vi "ROS_Master_Main.vi"(11 "ROS_Master in":refnum<class "ROS_Master.lvclass">) -> ()   [LabVIEW 2012, in "ROS_Master.lvclass"]
uses:
  <userlib>/ROSforLV/ROS/Code/ROS_Master/ROS_Master.lvclass
  <userlib>/ROSforLV/ROS/Code/ROS_Master/ROS_Master.lvclass/ROS_Master.ctl
  <userlib>/ROSforLV/ROS/Code/_ROSDefinition.vi
panel:
  in  "Port":u32=11311
  in  "stop":bool
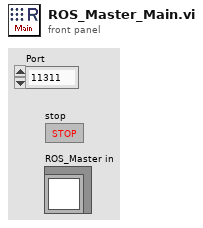
[diagram p1: front panel]
types:
  T1 = cluster{"Caller ID":string, "IP":string, "Msg Type":string, "Direction":enum16{"Publisher", "Subscriber"}, "Topic":string}
  T2 = cluster{"value":string, "value":string, "value":string}
  T3 = cluster{"Service":string, "Service IP":string, "Caller IP":string, "Caller ID":string}[]
  T4 = cluster{"Service":string, "Service IP":string, "Caller IP":string, "Caller ID":string}
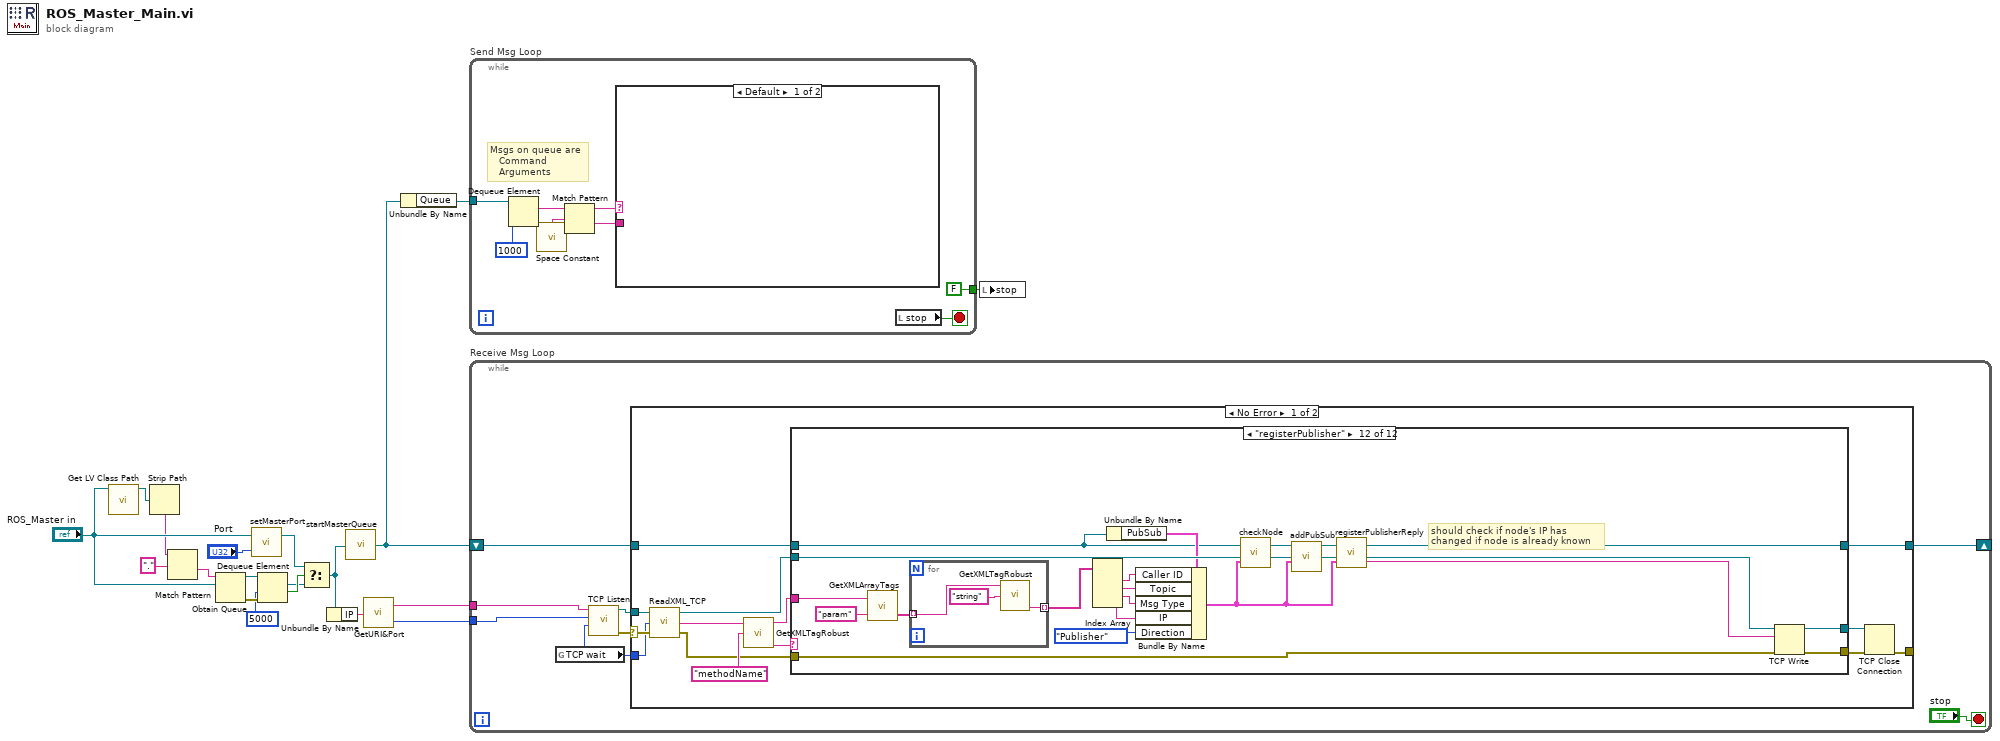
[diagram p0: block diagram]
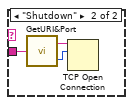
[diagram p2: hidden frame]
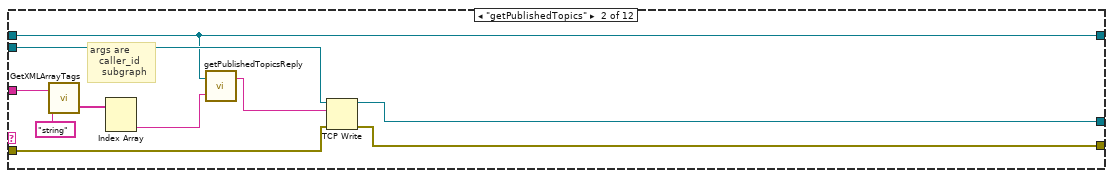
[diagram p4: hidden frame]
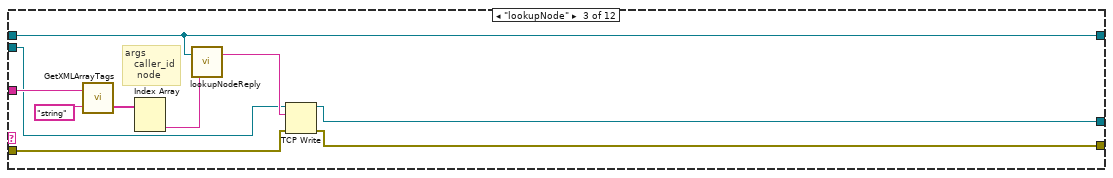
[diagram p5: hidden frame]
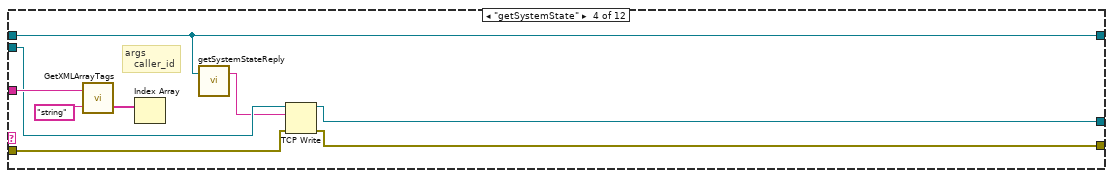
[diagram p6: hidden frame]
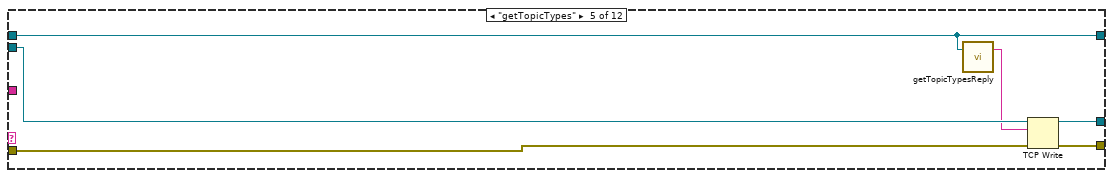
[diagram p7: hidden frame]
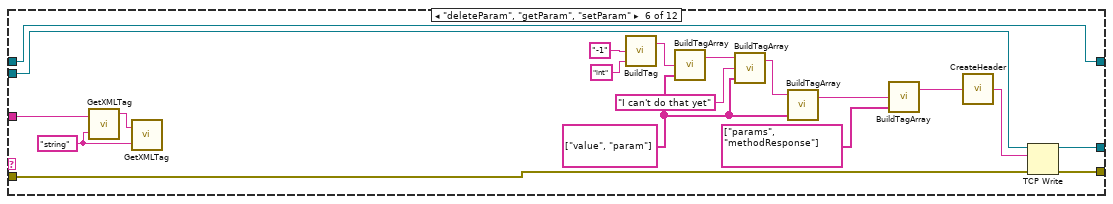
[diagram p8: hidden frame]
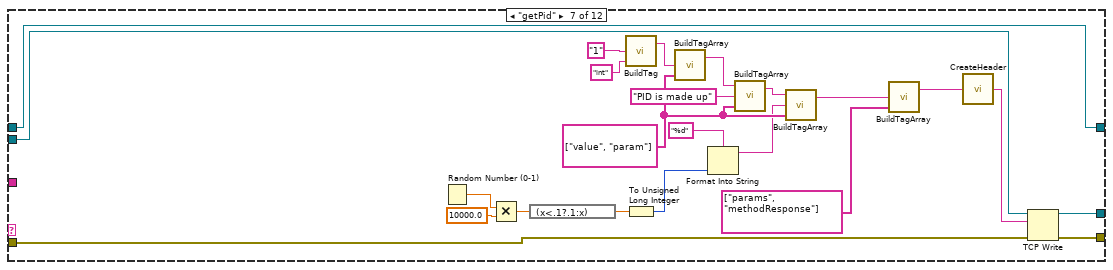
[diagram p9: hidden frame]
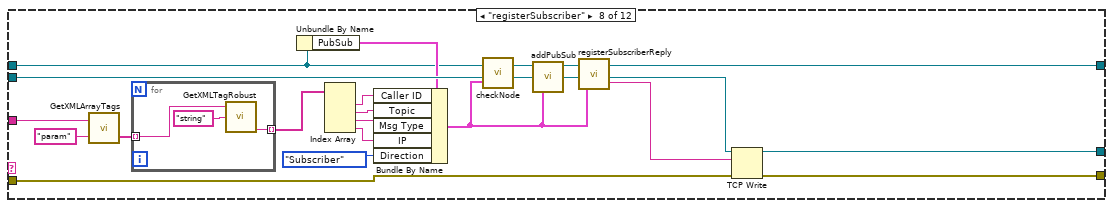
[diagram p10: hidden frame]
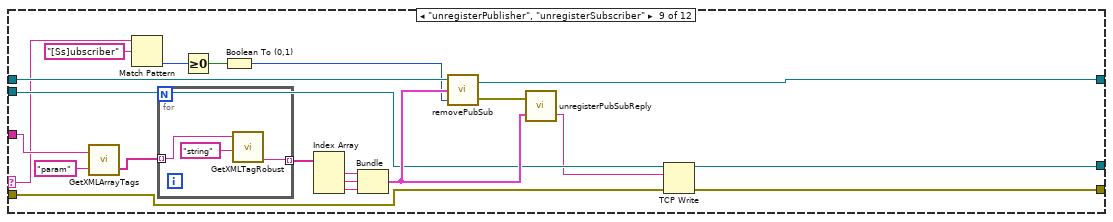
[diagram p11: hidden frame]
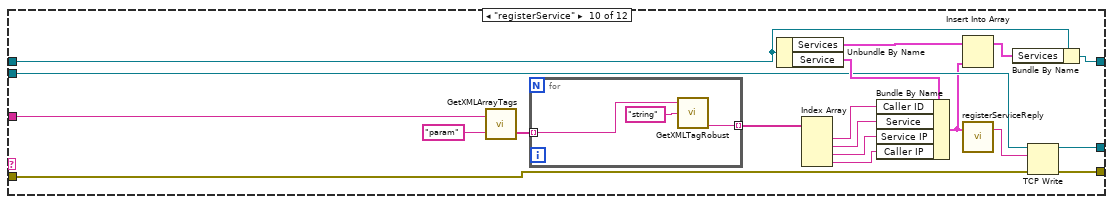
[diagram p12: hidden frame]
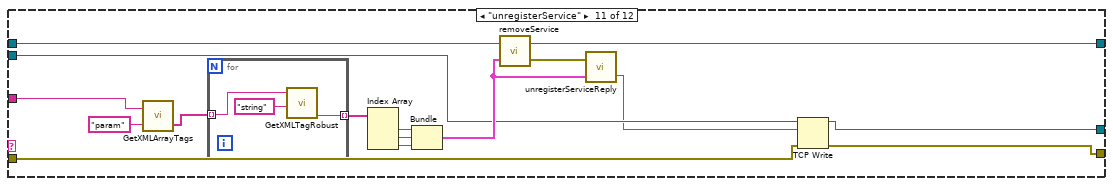
[diagram p13: hidden frame]
diagram:
  n1 = call <vilib>:"Get LV Class Path.vi"("object"="ROS_Master in") -> ("class path"=w3:path)  [unwired: 9 in, 1 out]
  n2 = Strip Path(path=w3) -> (name=w2:string)  [unwired: 1 out]
  n3 = Match Pattern(string=w2, regular expression=".") -> (after substring=w15:string)  [unwired: 1 in, 3 out]
  n4 = Obtain Queue(name (unnamed)=w15, element data type="ROS_Master in") -> (queue out=w13:refnum<queue>, error out=w14:errorcluster)  [unwired: 3 in, 1 out]
  n5 = call <userlib>:"setMasterPort.vi"("Port"="Port", "ROS_Master.lvclass in"="ROS_Master in") -> ("ROS_Master.lvclass out"=w10:refnum<class "ROS_Master.lvclass">)  [unwired: 1 in]
  n6 = Dequeue Element(queue=w13, timeout in ms (-1)=5000, error in (no error)=w14) -> (element=w9:refnum<class "ROS_Master.lvclass">, timed out?=w12:bool)  [unwired: 2 out]
  n7 = Select(t=w10, s=w12, f=w9) -> (s? t:f=w8:refnum<class "ROS_Master.lvclass">)
  n8 = Unbundle By Name(w8) -> ("IP"=w19:string)
  n9 = call <userlib>:"startMasterQueue.vi"("ROS_Master in"=w8) -> ("ROS_Master out"=w6:refnum<class "ROS_Master.lvclass">)
  n10 = call <userlib>:"GetURI&Port.vi"("URI in"=w19) -> ("Port"=w17:u16, "URI"=w18:string)
  n11 = Unbundle By Name(w6) -> ("Queue"=w5:refnum<queue>)
  n12 = while "Send Msg Loop" {
    tunnel: [FALSE ("stop")] -> w7
    tunnel: w5 -> [w25]
    stop <- w27 stop-if-true
    # "Msgs on queue are\n   Command\n   Arguments"
    n13 = Dequeue Element(queue=w25, timeout in ms (-1)=1000) -> (element=w23:string)  [unwired: 1 in, 3 out]
    n14 = call <vilib>:"Space Constant.vi"() -> ("String"=w22:string)
    n15 = Match Pattern(string=w23, regular expression=w22) -> (before substring=w21:string, after substring=w20:string)  [unwired: 1 in, 2 out]
    n16 = case shown="Default" w21 {
      tunnel: w20 -> [_ w30]
      frame Default {
      }
      frame "Shutdown" {
        n17 = call <userlib>:"GetURI&Port.vi"("URI in"=w30) -> ("Port"=w28:u16, "URI"=w29:string)
        n18 = TCP Open Connection(address=w29, remote port or service name=w28) -> ()  [unwired: 3 in, 2 out]
      }
    }
    n19 = local read "stop"() -> (w27:bool)
  }
  n20 = while "Receive Msg Loop" {
    shift-right: [w32] -> _
    shift-left: w6 -> [w33]
    tunnel: w18 -> [w36]
    tunnel: w17 -> [w35]
    stop <- "stop" stop-if-true
    n21 = global read "_ROSDefinition.vi" "TCP wait"() -> (w31:i32)
    n22 = call <vilib>:"TCP Listen.vi"("timeout ms (wait forever: -1)"=w31, "port"=w35, "service name"=w36) -> ("error out"=w37:errorcluster, "connection ID"=w34:refnum<k5>)  [unwired: 4 in, 3 out]
    n23 = case shown="No Error" w37 {
      selector: w37 -> [w51 _]
      tunnel: w34 -> [w52 _]
      tunnel: w33 -> [w46 w242]
      tunnel: [w45 w242] -> w32
      tunnel: w31 -> [w44 _]
      tunnel: [w39 _] -> _
      frame No Error {
        n24 = call <userlib>:"ReadXML_TCP.vi"("error in"=w51, "timeout ms (3000)"=w44, "connection ID in"=w52) -> ("error out"=w40:errorcluster, "data out"=w50:string, "connection ID out"=w43:refnum<k5>)
        n25 = call <userlib>:"GetXMLTagRobust.vi"("Tag"="methodName", "String"=w50) -> ("value"=w48:string, "String w/o Tag"=w47:string)  [unwired: 1 in, 2 out]
        n26 = case shown="\"registerPublisher\"" w48 {
          selector: w48 -> [_ _ _ _ _ _ _ _ w159 _ _ _]
          tunnel: w47 -> [_ w65 w75 w84 _ w108 _ w151 w175 w197 w212 w238]
          tunnel: w46 -> [w55 w56 w66 w77 w85 w109 w132 w134 w168 w193 w209 w222]
          tunnel: [w55 w56 w66 w77 w85 w109 w132 w142 w167 w187 w201 w229] -> w45
          tunnel: w43 -> [w54 w61 w70 w81 w88 w95 w119 w147 w163 w184 w206 w234]
          tunnel: [w54 w58 w67 w78 w90 w93 w118 w146 w161 w182 w203 w232] -> w42
          tunnel: [w53 w57 w68 w79 w89 w92 w117 w144 w160 w181 w202 w231] -> w41
          tunnel: w40 -> [w53 w59 w69 w80 w87 w94 w116 w145 w164 w183 w205 w233]
          frame Default {
          }
          frame "getPublishedTopics" {
            # "args are\n   caller_id\n    subgraph"
            n27 = call <userlib>:"GetXMLArrayTags.vi"("ArrayTag"="string", "String"=w65) -> ("Array"=w63:string[])  [unwired: 1 out]
            n28 = Index Array(array=w63) -> (element #2=w62:string)  [unwired: 2 in, 1 out]
            n29 = call <userlib>:"getPublishedTopicsReply.vi"("Subgraph"=w62, "ROS_Master"=w56) -> ("XML"=w60:string)  [unwired: 1 in]
            n30 = TCP Write(connection ID=w61, data in=w60, error in (no error)=w59) -> (connection ID out=w58:refnum<k5>, error out=w57:errorcluster)  [unwired: 1 in, 1 out]
          }
          frame "lookupNode" {
            # "args\n   caller_id\n    node"
            n31 = call <userlib>:"GetXMLArrayTags.vi"("ArrayTag"="string", "String"=w75) -> ("Array"=w73:string[])  [unwired: 1 out]
            n32 = Index Array(array=w73) -> (element #2=w72:string)  [unwired: 2 in, 1 out]
            n33 = call <userlib>:"lookupNodeReply.vi"("node"=w72, "Master"=w66) -> ("XML"=w71:string)  [unwired: 1 in]
            n34 = TCP Write(connection ID=w70, data in=w71, error in (no error)=w69) -> (connection ID out=w67:refnum<k5>, error out=w68:errorcluster)  [unwired: 1 in, 1 out]
          }
          frame "getSystemState" {
            # "args\n   caller_id"
            n35 = call <userlib>:"GetXMLArrayTags.vi"("ArrayTag"="string", "String"=w84) -> ("Array"=w82:string[])  [unwired: 1 out]
            n36 = Index Array(array=w82) -> ()  [unwired: 1 in, 1 out]
            n37 = call <userlib>:"getSystemStateReply.vi"("ROS_Master in"=w77) -> ("XML"=w76:string)  [unwired: 2 in]
            n38 = TCP Write(connection ID=w81, data in=w76, error in (no error)=w80) -> (connection ID out=w78:refnum<k5>, error out=w79:errorcluster)  [unwired: 1 in, 1 out]
          }
          frame "getTopicTypes" {
            n39 = call <userlib>:"getTopicTypesReply.vi"("ROS_Master.lvclass in"=w85) -> ("Topics XML"=w86:string)  [unwired: 2 in]
            n40 = TCP Write(connection ID=w88, data in=w86, error in (no error)=w87) -> (connection ID out=w90:refnum<k5>, error out=w89:errorcluster)  [unwired: 1 in, 1 out]
          }
          frame "deleteParam", "getParam", "setParam" {
            w105 = string[] ["value", "param"] ("tags")
            w106 = "string" ("Tag")
            n41 = call <userlib>:"GetXMLTag.vi"("Tag"=w106, "String"=w108) -> ("String w/o Tag"=w107:string)  [unwired: 2 out]
            n42 = call <userlib>:"GetXMLTag.vi"("Tag"=w106, "String"=w107) -> ()  [unwired: 3 out]
            n43 = call <userlib>:"BuildTag.vi"("tag"="int", "value"="-1") -> ("string out"=w99:string)  [unwired: 2 in]
            n44 = call <userlib>:"BuildTagArray.vi"("tags"=w105, "value"=w99) -> ("string out"=w104:string)  [unwired: 2 in]
            n45 = call <userlib>:"BuildTagArray.vi"("tags"=w105, "value"="I can't do that yet", "string in"=w104) -> ("string out"=w103:string)  [unwired: 1 in]
            n46 = call <userlib>:"BuildTagArray.vi"("tags"=w105, "string in"=w103) -> ("string out"=w97:string)  [unwired: 2 in]
            n47 = call <userlib>:"BuildTagArray.vi"("tags"=string[] ["params", "methodResponse"], "value"=w97) -> ("string out"=w96:string)  [unwired: 2 in]
            n48 = call <userlib>:"CreateHeader.vi"("Content"=w96) -> ("XML"=w91:string)
            n49 = TCP Write(connection ID=w95, data in=w91, error in (no error)=w94) -> (connection ID out=w93:refnum<k5>, error out=w92:errorcluster)  [unwired: 1 in, 1 out]
          }
          frame "getPid" {
            w131 = string[] ["value", "param"] ("tags")
            n50 = Random Number (0-1)() -> (number: 0 to 1=w128:dbl)
            n51 = Multiply(x=w128, y=10000.0) -> (x*y=w115:dbl)
            n52 = expression code="(x<.1?.1:x)"(w115) -> (w114:dbl)
            n53 = call <userlib>:"BuildTag.vi"("tag"="int", "value"="1") -> ("string out"=w110:string)  [unwired: 2 in]
            n54 = To Unsigned Long Integer(number=w114) -> (unsigned 32bit integer=w126:u32)
            n55 = call <userlib>:"BuildTagArray.vi"("tags"=w131, "value"=w110) -> ("string out"=w130:string)  [unwired: 2 in]
            n56 = Format Into String(format string="%d", w126) -> (resulting string=w124:string)  [unwired: 2 in, 1 out]
            n57 = call <userlib>:"BuildTagArray.vi"("tags"=w131, "value"="PID is made up", "string in"=w130) -> ("string out"=w129:string)  [unwired: 1 in]
            n58 = call <userlib>:"BuildTagArray.vi"("tags"=w131, "value"=w124, "string in"=w129) -> ("string out"=w123:string)  [unwired: 1 in]
            n59 = call <userlib>:"BuildTagArray.vi"("tags"=string[] ["params", "methodResponse"], "value"=w123) -> ("string out"=w121:string)  [unwired: 2 in]
            n60 = call <userlib>:"CreateHeader.vi"("Content"=w121) -> ("XML"=w120:string)
            n61 = TCP Write(connection ID=w119, data in=w120, error in (no error)=w116) -> (connection ID out=w118:refnum<k5>, error out=w117:errorcluster)  [unwired: 1 in, 1 out]
          }
          frame "registerSubscriber" {
            n62 = call <userlib>:"GetXMLArrayTags.vi"("ArrayTag"="param", "String"=w151) -> ("Array"=w149:string[])  [unwired: 1 out]
            n63 = for {
              tunnel: w149 -> [w154] mode=indexing
              tunnel: [w152] -> w148 mode=indexing
              n64 = call <userlib>:"GetXMLTagRobust.vi"("Tag"="string", "String"=w154) -> ("value"=w152:string)  [unwired: 1 in, 3 out]
            }
            n65 = Unbundle By Name(w134) -> ("PubSub"=w137:T1)
            n66 = Index Array(array=w148) -> (element #1=w141:string, element #2=w140:string, element #3=w139:string, element #4=w138:string)  [unwired: 4 in]
            n67 = Bundle By Name(cluster=w137, "Caller ID"=w141, "Topic"=w140, "Msg Type"=w139, "IP"=w138, "Direction"=enum16{"Publisher", "Subscriber"}."Subscriber") -> (w135:T1)
            n68 = call <userlib>:"checkNode.vi"("PubSub"=w135, "ROS_Master"=w134) -> ("ROS_Master out"=w133:refnum<class "ROS_Master.lvclass">)  [unwired: 1 in]
            n69 = call <userlib>:"addPubSub.vi"("PubSub"=w135, "ROS_Master in"=w133) -> ("ROS_Master out"=w142:refnum<class "ROS_Master.lvclass">)  [unwired: 9 in]
            n70 = call <userlib>:"registerSubscriberReply.vi"("Subscriber"=w135, "ROS_Master.lvclass in"=w142) -> ("XML"=w143:string)  [unwired: 1 in]
            n71 = TCP Write(connection ID=w147, data in=w143, error in (no error)=w145) -> (connection ID out=w146:refnum<k5>, error out=w144:errorcluster)  [unwired: 1 in, 1 out]
          }
          frame "unregisterPublisher", "unregisterSubscriber" {
            n72 = call <userlib>:"GetXMLArrayTags.vi"("ArrayTag"="param", "String"=w175) -> ("Array"=w173:string[])  [unwired: 1 out]
            n73 = Match Pattern(string=w159, regular expression="[Ss]ubscriber") -> (offset past match=w157:i32)  [unwired: 1 in, 3 out]
            n74 = for {
              tunnel: w173 -> [w178] mode=indexing
              tunnel: [w176] -> w172 mode=indexing
              n75 = call <userlib>:"GetXMLTagRobust.vi"("Tag"="string", "String"=w178) -> ("value"=w176:string)  [unwired: 1 in, 3 out]
            }
            n76 = Greater Or Equal To 0?(x=w157) -> (x >= 0?=w156:bool)
            n77 = Boolean To (0,1)(Boolean=w156) -> (0, 1=w155:i16)
            n78 = Index Array(array=w172) -> (element #1=w171:string, element #2=w170:string, element #3=w169:string)  [unwired: 3 in]
            n79 = Bundle("value"=w171, "value"=w170, "value"=w169) -> (w166:T2)  [unwired: 1 in]
            n80 = call <userlib>:"removePubSub.vi"("Direction"=w155, "PubSub"=w166, "ROS_Master in"=w168) -> ("error out"=w165:errorcluster, "ROS_Master out"=w167:refnum<class "ROS_Master.lvclass">)
            n81 = call <userlib>:"unregisterPubSubReply.vi"("PubSub"=w166, "error in"=w165) -> ("XML"=w162:string)  [unwired: 1 in]
            n82 = TCP Write(connection ID=w163, data in=w162, error in (no error)=w164) -> (connection ID out=w161:refnum<k5>, error out=w160:errorcluster)  [unwired: 1 in, 1 out]
          }
          frame "registerService" {
            n83 = call <userlib>:"GetXMLArrayTags.vi"("ArrayTag"="param", "String"=w197) -> ("Array"=w195:string[])  [unwired: 1 out]
            n84 = for {
              tunnel: w195 -> [w200] mode=indexing
              tunnel: [w198] -> w194 mode=indexing
              n85 = call <userlib>:"GetXMLTagRobust.vi"("Tag"="string", "String"=w200) -> ("value"=w198:string)  [unwired: 1 in, 3 out]
            }
            n86 = Unbundle By Name(w193) -> ("Services"=w188:T3, "Service"=w192:T4)
            n87 = Index Array(array=w194) -> (element #1=w191:string, element #2=w190:string, element #3=w189:string, element #4=w186:string)  [unwired: 4 in]
            n88 = Bundle By Name(cluster=w192, "Caller ID"=w191, "Service"=w190, "Service IP"=w189, "Caller IP"=w186) -> (w180:T4)
            n89 = Insert Into Array(array=w188, new element=w180) -> (w185:T3)  [unwired: 1 in]
            n90 = call <userlib>:"registerServiceReply.vi"("Service"=w180) -> ("XML"=w179:string)  [unwired: 2 in]
            n91 = Bundle By Name(cluster=w193, "Services"=w185) -> (w187:refnum<class "ROS_Master.lvclass">)
            n92 = TCP Write(connection ID=w184, data in=w179, error in (no error)=w183) -> (connection ID out=w182:refnum<k5>, error out=w181:errorcluster)  [unwired: 1 in, 1 out]
          }
          frame "unregisterService" {
            n93 = call <userlib>:"GetXMLArrayTags.vi"("ArrayTag"="param", "String"=w212) -> ("Array"=w211:string[])  [unwired: 1 out]
            n94 = for {
              tunnel: w211 -> [w218] mode=indexing
              tunnel: [w217] -> w210 mode=indexing
              n95 = call <userlib>:"GetXMLTagRobust.vi"("Tag"="string", "String"=w218) -> ("value"=w217:string)  [unwired: 1 in, 3 out]
            }
            n96 = Index Array(array=w210) -> (element #1=w215:string, element #2=w214:string, element #3=w213:string)  [unwired: 3 in]
            n97 = Bundle("value"=w215, "value"=w214, "value"=w213) -> (w207:T2)  [unwired: 1 in]
            n98 = call <userlib>:"removeService.vi"("Service"=w207, "ROS_Master in"=w209) -> ("error out"=w208:errorcluster, "ROS_Master out"=w201:refnum<class "ROS_Master.lvclass">)
            n99 = call <userlib>:"unregisterServiceReply.vi"("Service"=w207, "error in"=w208) -> ("XML"=w204:string)  [unwired: 1 in]
            n100 = TCP Write(connection ID=w206, data in=w204, error in (no error)=w205) -> (connection ID out=w203:refnum<k5>, error out=w202:errorcluster)  [unwired: 1 in, 1 out]
          }
          frame "registerPublisher" {
            # "should check if node's IP has \nchanged if node is already known"
            n101 = call <userlib>:"GetXMLArrayTags.vi"("ArrayTag"="param", "String"=w238) -> ("Array"=w236:string[])  [unwired: 1 out]
            n102 = for {
              tunnel: w236 -> [w241] mode=indexing
              tunnel: [w239] -> w235 mode=indexing
              n103 = call <userlib>:"GetXMLTagRobust.vi"("Tag"="string", "String"=w241) -> ("value"=w239:string)  [unwired: 1 in, 3 out]
            }
            n104 = Index Array(array=w235) -> (element #1=w228:string, element #2=w227:string, element #3=w226:string, element #4=w225:string)  [unwired: 4 in]
            n105 = Unbundle By Name(w222) -> ("PubSub"=w224:T1)
            n106 = Bundle By Name(cluster=w224, "Caller ID"=w228, "Topic"=w227, "Msg Type"=w226, "IP"=w225, "Direction"=enum16{"Publisher", "Subscriber"}."Publisher") -> (w221:T1)
            n107 = call <userlib>:"checkNode.vi"("PubSub"=w221, "ROS_Master"=w222) -> ("ROS_Master out"=w220:refnum<class "ROS_Master.lvclass">)  [unwired: 1 in]
            n108 = call <userlib>:"addPubSub.vi"("PubSub"=w221, "ROS_Master in"=w220) -> ("ROS_Master out"=w229:refnum<class "ROS_Master.lvclass">)  [unwired: 9 in]
            n109 = call <userlib>:"registerPublisherReply.vi"("Publisher"=w221, "ROS_Master.lvclass in"=w229) -> ("XML"=w230:string)  [unwired: 1 in]
            n110 = TCP Write(connection ID=w234, data in=w230, error in (no error)=w233) -> (connection ID out=w232:refnum<k5>, error out=w231:errorcluster)  [unwired: 1 in, 1 out]
          }
        }
        n111 = TCP Close Connection(connection ID=w42, error in (no error)=w41) -> (error out=w39:errorcluster)  [unwired: 1 in, 1 out]
      }
      frame Error {
      }
    }
  }
  n112 = local write "stop"(w7) -> ()
